vi "Send Add Client.vi"(6 "Service Name":string, 7 "Priority":T1=enum."Normal" caption="Message Priority (Normal)", 8 "error in (no error)":errorcluster, 9 "Client ID":string, 10 "WebSocket Connection":refnum<k5>, 11 "Message Enqueuer in":refnum<class "Message Enqueuer.lvclass">) -> (0 "error out":errorcluster, 3 "Message Enqueuer out":refnum<class "Message Enqueuer.lvclass">)   [LabVIEW 2021, in "WebSocket Actors.lvlib" / "Add Client Msg.lvclass"]
doc: "Sends the <b>WebSocket Actors.lvlib:Add Client Msg.lvclass</b> message.\n\nThis message will call <b>Add Client.vi</b> on the <b>WebSocket Actors.lvlib:WebSocket Service.lvclass</b> actor.\n\n<b>Add Client.vi Description</b>\nThe WebSocket server has successfully completed the handshake and accepted client connection. This method starts the WebSocket Connection actor that will handle the communication to this particular client connected to this service"
uses:
  Add Client Msg.lvclass
  Add Client Msg.lvclass/Add Client Msg.ctl
  <vilib>/ActorFramework/Message Enqueuer/Message Enqueuer.lvclass
  C:/Program Files/National Instruments/LabVIEW 2021/vi.lib/ActorFramework/Message/Message.lvclass
  C:/Projects/WebSocket-Actor/WebSocket Actor/WebSocket Service Messages/Add Client Msg/Add Client Msg.lvclass
  <vilib>/ActorFramework/Message Enqueuer/Message Priority.ctl
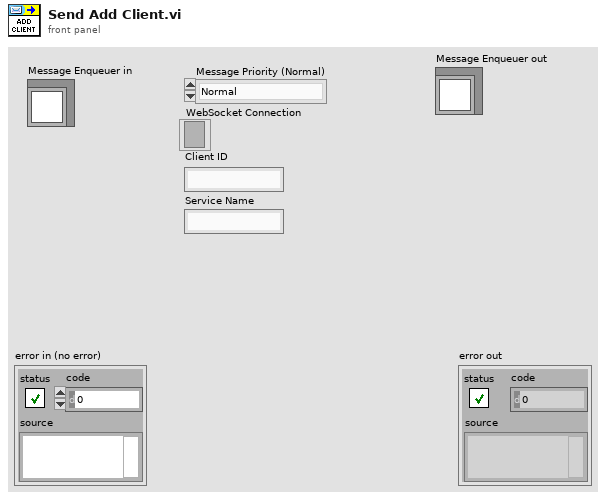
[diagram p1: front panel]
types:
  T1 = typedef "Actor Framework.lvlib/Message Enqueuer.lvclass/Message Priority.ctl" = enum16{"Low", "Normal", "High"}
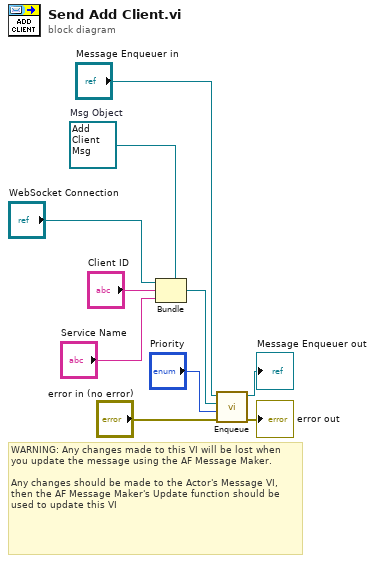
[diagram p0: block diagram]
diagram:
  w7 = refnum<class "Add Client Msg.lvclass"> refnum  # Msg Object
  # "WARNING: Any changes made to this VI will be lost when you update the message using the AF Message Maker.\n\nAny changes should be made to the Actor's Message VI, then the AF Message Maker's Update function should be used to update this VI"
  n1 = Bundle(cluster=w7, "WebSocket Connection", "Client ID", "Service Name") -> (w2:refnum<class "Add Client Msg.lvclass">)
  n2 = call <vilib>:"Enqueue.vi"("error in (no error)"="error in (no error)", "Message Priority (Normal)"="Priority", "Message"=w2, "Message Enqueuer in"="Message Enqueuer in") -> ("error out"=→"error out":errorcluster, "Message Enqueuer out"=→"Message Enqueuer out":refnum<class "Message Enqueuer.lvclass">)  [unwired: 6 in]
